vi "Periodic Tasks.vi"(8 "error in":errorcluster) -> ()   [LabVIEW 2016]
doc: "This VI runs in parallel to other tasks. It can contain as many user-defined periodic loops as you need. These can carry out PID or other sorts of timed response."
uses:
  Control Files/Extra Motors.ctl
  Robot Global Data.vi
  Control Files/DriveMotors.ctl
  Control Files/SwerveMotors.ctl
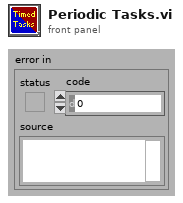
[diagram p1: front panel]
types:
  T1 = typedef "SwerveMotors.ctl" = enum16{"Swerve 1", "Swerve 2", "Swerve 3", "Swerve 4"}
  T2 = typedef "DriveMotors.ctl" = enum16{"Drive1", "Drive2", "Drive3", "Drive4"}
  T3 = typedef "Extra Motors.ctl" = enum16{"Climber"}
  T4 = typedef "WPI_MotorControlDeviceRef.ctl" = cluster{"DeviceStatus":errorcluster, "Type":T5, "PWM":cluster{"PWM Channel":T6, "DeadBand":T7}, "CAN":cluster{"Device Number":u8, "SetOutput VI Ref":variant, "GetOutput VI Ref":variant, "Enable VI Ref":variant, "Disable VI Ref":variant, "Data":variant}, "Invert":bool}
  T5 = typedef "WPI_MotorControlType.ctl" = enum16{"PWM", "CAN"}
  T6 = typedef "FPGA_DIOPWMChannel.ctl" = enum8{"PWM 0", "PWM 1", "PWM 2", "PWM 3", "PWM 4", "PWM 5", "PWM 6", "PWM 7", "PWM 8", "PWM 9", "PWM MXP 0", "PWM MXP 1", "PWM MXP 2", "PWM MXP 3", "PWM MXP 4", "PWM MXP 5", "PWM MXP 6", "PWM MXP 7", "PWM MXP 8", "PWM MXP 9", "Invalid"}
  T7 = typedef "WPI_PWMDeadband.ctl" = cluster{"Name":string, "maxPositivePwm":i32, "minPositivePwm":i32, "centerPwm":i32, "maxNegativePwm":i32, "minNegativePwm":i32, "angularRange":u16}
  T8 = cluster{"X":dbl, "Y":dbl, "Z":dbl, "B (Straight Drive)":bool, "T1 Climber Up":bool}
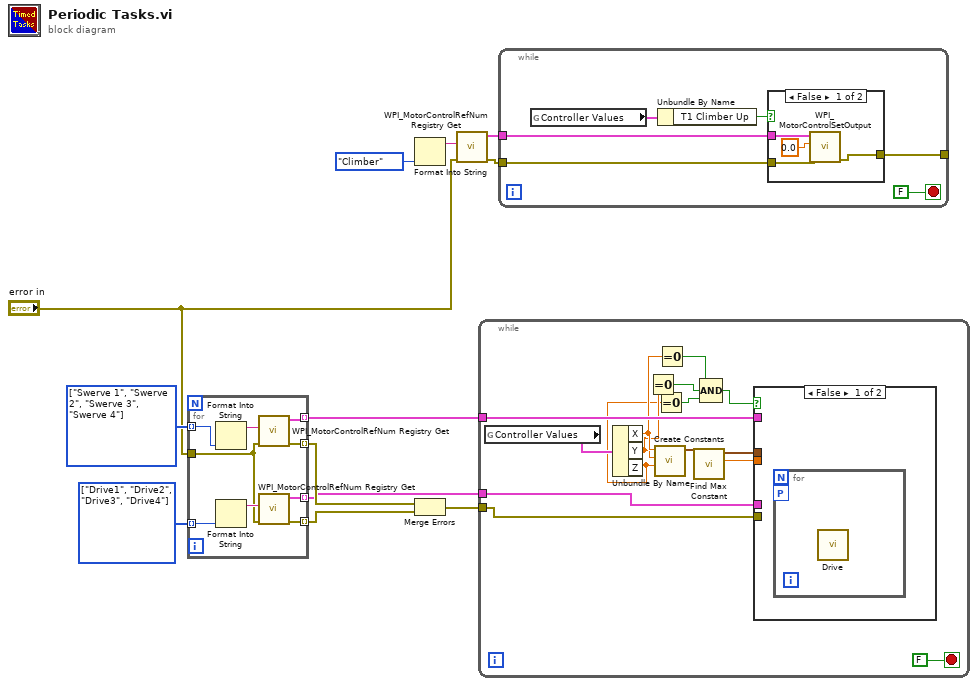
[diagram p0: block diagram]
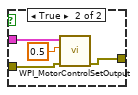
[diagram p3: hidden frame]
diagram:
  w7 = T1[] [enum."Swerve 1", enum."Swerve 2", enum."Swerve 3", enum."Swerve 4"] items=["Swerve 1", "Swerve 2", "Swerve 3", "Swerve 4"] ("Array")
  w8 = T2[] [enum."Drive1", enum."Drive2", enum."Drive3", enum."Drive4"] items=["Drive1", "Drive2", "Drive3", "Drive4"] ("Array")
  n1 = for {
    tunnel: w8 -> [w21] mode=indexing
    tunnel: w7 -> [w20] mode=indexing
    tunnel: "error in" -> [w17]
    tunnel: [w16] -> w5 mode=indexing
    tunnel: [w15] -> w4 mode=indexing
    tunnel: [w14] -> w2 mode=indexing
    tunnel: [w13] -> w1 mode=indexing
    n2 = Format Into String(w20) -> (resulting string=w19:string)  [unwired: 3 in, 1 out]
    n3 = Format Into String(w21) -> (resulting string=w18:string)  [unwired: 3 in, 1 out]
    n4 = call <vilib>:"WPI_MotorControlRefNum Registry Get.vi"("error in (no error)"=w17, "refnum name"=w19) -> ("error out"=w15:errorcluster, "MotorControlDevRef"=w14:T4)  [unwired: 8 in]
    n5 = call <vilib>:"WPI_MotorControlRefNum Registry Get.vi"("error in (no error)"=w17, "refnum name"=w18) -> ("error out"=w16:errorcluster, "MotorControlDevRef"=w13:T4)  [unwired: 8 in]
  }
  n6 = Format Into String(Extra_Motors."Climber" ("Enum")) -> (resulting string=w11:string)  [unwired: 3 in, 1 out]
  n7 = Merge Errors(w4, w5) -> (w3:errorcluster)
  n8 = call <vilib>:"WPI_MotorControlRefNum Registry Get.vi"("error in (no error)"="error in", "refnum name"=w11) -> ("error out"=w9:errorcluster, "MotorControlDevRef"=w10:T4)  [unwired: 8 in]
  n9 = while {
    tunnel: w3 -> [w29]
    tunnel: w2 -> [w31]
    tunnel: w1 -> [w30]
    stop <- FALSE stop-if-true
    n10 = global read "Robot Global Data.vi" "Controller Values"() -> (w35:T8)
    n11 = Unbundle By Name(w35) -> ("X"=w24:dbl, "Y"=w23:dbl, "Z"=w22:dbl)
    n12 = Equal To 0?(x=w23) -> (x = 0?=w27:bool)
    n13 = call "Create Constants.vi"("Z"=w22, "Y"=w23, "X"=w24) -> ("constants cluster"=w34:cluster{"a":dbl, "b":dbl, "c":dbl, "d":dbl})  [unwired: 8 in]
    n14 = Equal To 0?(x=w22) -> (x = 0?=w26:bool)
    n15 = Equal To 0?(x=w24) -> (x = 0?=w28:bool)
    n16 = call "Find Max Constant.vi"("constants in"=w34) -> ("Max or 1"=w32:dbl, "constants out"=w33:cluster{"a":dbl, "b":dbl, "c":dbl, "d":dbl})  [unwired: 9 in]
    n17 = Compound Arithmetic op=AND(w28, w27, w26) -> (w25:bool)
    n18 = case shown="False" w25 {
      tunnel: w33 -> [_ w41]
      tunnel: w32 -> [_ w40]
      tunnel: w31 -> [_ w39]
      tunnel: w30 -> [_ w38]
      tunnel: w29 -> [_ w37]
      frame False {
        n19 = for {
          workers-P: _ -> [_]
          n20 = call "Drive.vi"() -> ()  [unwired: 12 in]
        }
      }
      frame True {
        n21 = for {
          tunnel: w41 -> [_]
          tunnel: w40 -> [_]
          tunnel: w39 -> [_] mode=indexing
          tunnel: w38 -> [_] mode=indexing
          workers-P: _ -> [_]
          tunnel: w37 -> [_]
        }
      }
    }
  }
  n22 = while {
    tunnel: w10 -> [w47]
    tunnel: w9 -> [w44]
    tunnel: [w43] -> _
    stop <- FALSE stop-if-true
    n23 = global read "Robot Global Data.vi" "Controller Values"() -> (w46:T8)
    n24 = Unbundle By Name(w46) -> ("T1 Climber Up"=w45:bool)
    n25 = case shown="False" w45 {
      tunnel: w47 -> [w51 w55]
      tunnel: w44 -> [w49 w53]
      tunnel: [w48 w52] -> w43
      frame False {
        n26 = call <vilib>:"WPI_MotorControlSetOutput.vi"("error in (no error)"=w49, "Output"=0.0, "MotorControlDevRef"=w51) -> ("error out"=w48:errorcluster)  [unwired: 6 in, 2 out]
      }
      frame True {
        n27 = call <vilib>:"WPI_MotorControlSetOutput.vi"("error in (no error)"=w53, "Output"=0.5, "MotorControlDevRef"=w55) -> ("error out"=w52:errorcluster)  [unwired: 6 in, 2 out]
      }
    }
  }
